vi "LCB Read Event Ex.vi"(8 "error in (no error)":errorcluster caption="Fehler (Eingang, kein Fehler)") -> (0 "error out":errorcluster caption="Fehler (Ausgang)", 3 "Event Data":T1)   [LabVIEW 2010, in "labbCAN_Bus_API.lvlib"]
doc: "LCB_Func long __stdcall LCB_ReadEvent(long *pEventId,\n long *pData1,\n long *pData2,\n long *pData3);"
uses:
  labbCAN_Bus_API.lvlib
  labbCAN_Bus_API.dll
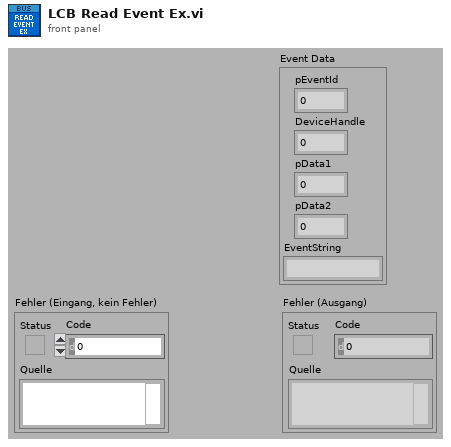
[diagram p1: front panel]
types:
  T1 = cluster{"pEventId":i32, "DeviceHandle":i64, "pData1":i32, "pData2":i32, "EventString":string}
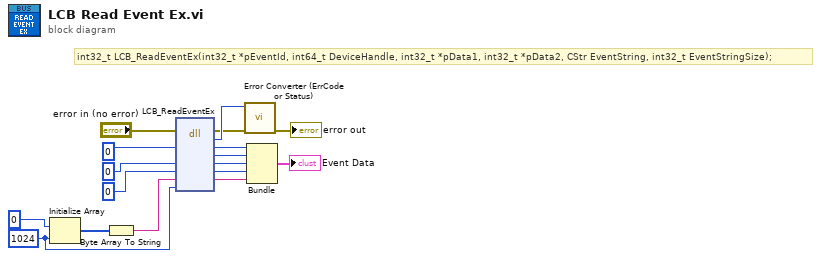
[diagram p0: block diagram]
diagram:
  w1 = 1024 ("Dimension")
  # "int32_t LCB_ReadEventEx(int32_t *pEventId, int64_t DeviceHandle, int32_t *pData1, int32_t *pData2, CStr EventString, int32_t EventStringSize);"
  n1 = Initialize Array(u8 0 ("Element"), w1) -> (w4:u8[])
  n2 = Byte Array To String(unsigned byte array=w4) -> (string=w2:string)
  n3 = dll-call lib="C:/CodingXP/cetoni_projects/QmixSDK/labbCAN_Bus_API.*" fn="LCB_ReadEventEx"(error in="error in (no error)", "pEventId"=0, "pData1"=0, "pData2"=0, "EventString"=w2, "EventStringSize"=w1) -> (error out=w12:errorcluster, "Rückgabetyp"=w13:i32, "pEventId"=w10:i32, "DeviceHandle"=w9:i64, "pData1"=w8:i32, "pData2"=w7:i32, "EventString"=w6:string)  [unwired: 4 in, 1 out]
  n4 = call "Error Converter (ErrCode or Status).vi"("error in (no error)"=w12, "error code"=w13) -> ("error out"=→"error out":errorcluster)  [unwired: 9 in]
  n5 = Bundle("pEventId"=w10, "DeviceHandle"=w9, "pData1"=w8, "pData2"=w7, "EventString"=w6) -> (→"Event Data":T1)  [unwired: 1 in]
